vi "Radoslaw_Wolnik_3.1.vi"() -> ()   [LabVIEW 2020]
panel:
  in  "stop":bool
  out "Losowa liczba":i8
  # "Program generuje losową liczbę w zakresie od 0 do 100 co 5s"
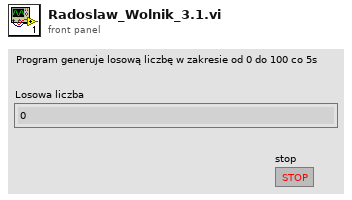
[diagram p1: front panel]
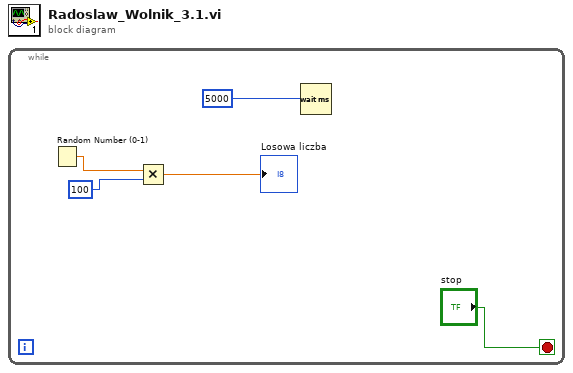
[diagram p0: block diagram]
diagram:
  n1 = while {
    stop <- "stop" stop-if-true
    n2 = Random Number (0-1)() -> (number: 0 to 1=w4:dbl)
    n3 = Multiply(x=w4, y=100) -> (x*y=→"Losowa liczba":dbl)
    n4 = Wait (ms)(milliseconds to wait=5000) -> ()  [unwired: 1 out]
  }
